vi "Copy file to network and group server.vi"(11 "File path in":path) -> ()   [LabVIEW 2011]
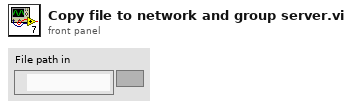
[diagram p1: front panel]
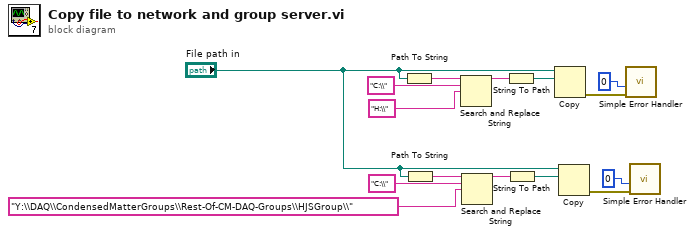
[diagram p0: block diagram]
diagram:
  n1 = Path To String(path="File path in") -> (string=w14:string)
  n2 = Path To String(path="File path in") -> (string=w9:string)
  n3 = Search and Replace String(input string=w14, search string="C:\\", replace string="H:\\") -> (result string=w15:string)  [unwired: 5 in, 3 out]
  n4 = Search and Replace String(input string=w9, search string="C:\\", replace string="Y:\\DAQ\\CondensedMatterGroups\\Rest-Of-CM-DAQ-Groups\\HJSGroup\\") -> (result string=w11:string)  [unwired: 5 in, 3 out]
  n5 = String To Path(string=w15) -> (path=w1:path)
  n6 = String To Path(string=w11) -> (path=w10:path)
  n7 = Copy(10:w1, 11:"File path in") -> (0:w5:errorcluster)  [unwired: 3 in, 2 out]
  n8 = Copy(10:w10, 11:"File path in") -> (0:w3:errorcluster)  [unwired: 3 in, 2 out]
  n9 = call <vilib>:"Simple Error Handler.vi"("type of dialog (OK msg:1)"=0, "error in (no error)"=w5) -> ()  [unwired: 3 in, 5 out]
  n10 = call <vilib>:"Simple Error Handler.vi"("type of dialog (OK msg:1)"=0, "error in (no error)"=w3) -> ()  [unwired: 3 in, 5 out]
